vi "NEXT TEMP.vi"(8 "error in (no error)":errorcluster, 9 "Boolean":bool, 10 "SweepQ":refnum<queue>, 11 "TempQ":refnum<queue>) -> (0 "error out":errorcluster, 2 "SweepQ Out":refnum<queue>, 3 "TEMPQ Out":refnum<queue>)   [LabVIEW 2025]
uses:
  TEMP_SWEEPER.ctl
  Temp Cntrl.ctl
  <userlib>/Nanonis Prog Interface V5e/Nanonis Prog Interface.lvlib
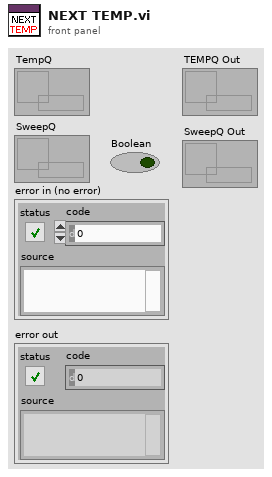
[diagram p1: front panel]
types:
  T1 = enum16{"SET TEMP", "SWEEP IDLE", "NEXT TEMP", "SWEEP DONE"}
  T2 = typedef "TEMP_SWEEPER.ctl" = cluster{"Temps(K)":dbl[], "Sweep States":enum16{"SET TEMP", "SWEEP IDLE", "NEXT TEMP", "SWEEP DONE"}}
  T3 = enum16{"1. INIT TEMP", "2. TC ON", "3. POLL_TEMPS", "4. TEMP_STAB", "5. TC IDLE", "6. APPLY NEXT TEMP", "7. TC OFF (Reset)"}
  T4 = typedef "Temp Cntrl.ctl" = cluster{"Range (0:Off)":u16, "Manual Output (0.00 %)":dbl, "Rate (D) (0.0 %)":dbl, "Reset (I) (20.0)":dbl, "Gain (P) (50.0)":dbl, "Power Up Enable (F: Disable)":bool, "Max User Current (2.000)":dbl, "Heater Resistance (1:25 Ohms)":u16, "Max Current (0:User Specified)":u16, "Heater Out Display (1:Current)":u16, "Mode (0:Off)":u16, "Input (0:None)":u16, "Target Temp (K)":dbl, "Serial Configuration":cluster{"Baud Rate":u32, "Parity":u16, "Data Bits":u16, "Stop Bits":u16, "Flow Control":u16}, "VISA resource name":refnum<visa-resource-name>, "Configure Control Parameters (0: Configure)":u16, "Enable Setpoint (F:Disable)":bool, "Input (0:A)":u16, "Data Source (0:Kelvin)":u16, "Output's Control Loop (1:1)":u16, "STND DEV Threshold ":dbl, "Mean Tolerance ":dbl, "Current State":enum16{"1. INIT TEMP", "2. TC ON", "3. POLL_TEMPS", "4. TEMP_STAB", "5. TC IDLE", "6. APPLY NEXT TEMP", "7. TC OFF (Reset)"}}
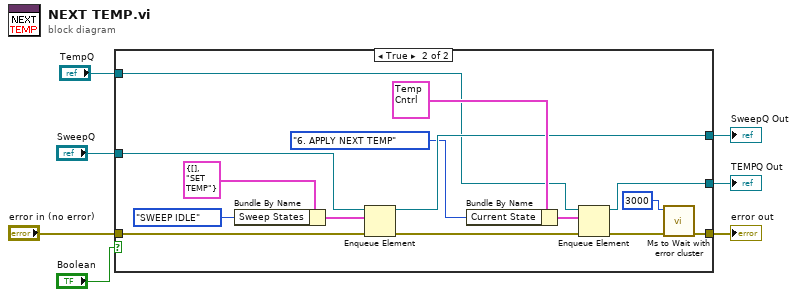
[diagram p0: block diagram]
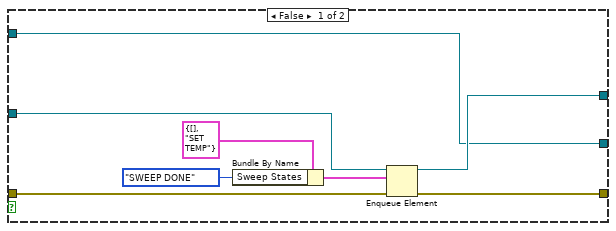
[diagram p2: hidden frame]
diagram:
  n1 = case shown="True" "Boolean" {
    tunnel: "SweepQ" -> [w12 w28]
    tunnel: "error in (no error)" -> [w11 w25]
    tunnel: [w10 w16] -> w4
    tunnel: [w9 w23] -> w1
    tunnel: [w13 w22] -> w3
    tunnel: "TempQ" -> [w9 w21]
    frame False {
      n2 = Bundle By Name(cluster=T2 {"Temps(K)"=[], "Sweep States"=enum."SET TEMP"} ("Temp and Field Range"), "Sweep States"=T1."SWEEP DONE") -> (w14:T2)
      n3 = Enqueue Element(queue=w12, element=w14, error in (no error)=w11) -> (queue out=w13:refnum<queue>, error out=w10:errorcluster)  [unwired: 1 in, 1 out]
    }
    frame True {
      n4 = Bundle By Name(cluster=T2 {"Temps(K)"=[], "Sweep States"=enum."SET TEMP"} ("Temp and Field Range"), "Sweep States"=T1."SWEEP IDLE") -> (w29:T2)
      n5 = Enqueue Element(queue=w28, element=w29, error in (no error)=w25) -> (queue out=w22:refnum<queue>, error out=w24:errorcluster)  [unwired: 1 in, 1 out]
      n6 = Bundle By Name(cluster=T4 {"Range (0:Off)"=0, "Manual Output (0.00 %)"=0.0, "Rate (D) (0.0 %)"=0.0, "Reset (I) (20.0)"=20.0, "Gain (P) (50.0)"=50.0, "Power Up Enable (F: Disable)"=FALSE, "Max User Current (2.000)"=2.0, "Heater Resistance (1:25 Ohms)"=1, "Max Current (0:User Specified)"=0, "Heater Out Display (1:Current)"=1, "Mode (0:Off)"=1, "Input (0:None)"=4, "Target Temp (K)"=5.0, "Serial Configuration"={"Baud Rate"=57600, "Parity"=1, "Data Bits"=7, "Stop Bits"=10, "Flow Control"=0}, "VISA resource name"="", "Configure Control Parameters (0: Configure)"=0, "Enable Setpoint (F:Disable)"=FALSE, "Input (0:A)"=3, "Data Source (0:Kelvin)"=0, "Output's Control Loop (1:1)"=2, "STND DEV Threshold "=0.1, "Mean Tolerance "=0.02, "Current State"=enum."1. INIT TEMP"} ("element"), "Current State"=T3."6. APPLY NEXT TEMP") -> (w26:T4)
      n7 = Enqueue Element(queue=w21, element=w26, error in (no error)=w24) -> (queue out=w23:refnum<queue>, error out=w17:errorcluster)  [unwired: 1 in, 1 out]
      n8 = call <userlib>:"Ms to Wait with error cluster.vi"("error in (no error)"=w17, "milliseconds to wait"=u32 3000) -> ("error out"=w16:errorcluster)  [unwired: 4 in, 1 out]
    }
  }
  "error out" <- w4
  "TEMPQ Out" <- w1
  "SweepQ Out" <- w3
